vi "p2.vi"() -> ()   [LabVIEW 2023, in "d12.lvlib"]
uses:
  d12.lvlib
  AOC/AOC.lvlib
panel:
  out "Answer":u64=7670
  in  "Example":string="???.### 1,1,3\n.??..??...?##. 1,1,3\n?#?#?#?#?#?#?#? 1,3,1,6\n????.#...#... 4,1,1\n????.######..#####. 1,6,5\n?###???????? 3,2,1"
  in  "Example":bool
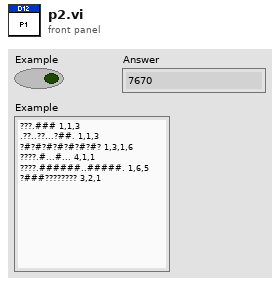
[diagram p1: front panel]
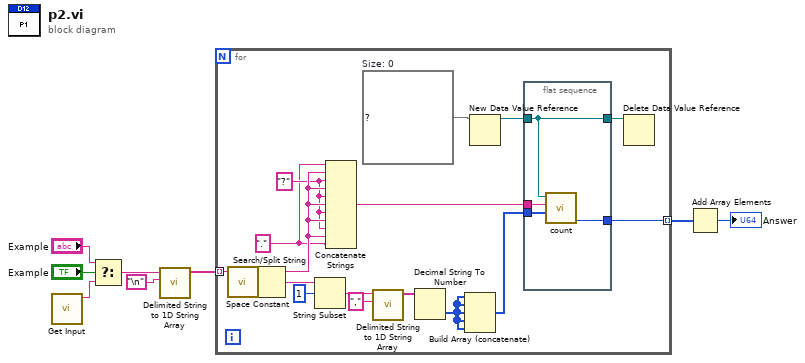
[diagram p0: block diagram]
diagram:
  n1 = call "Get Input.vi"() -> ("Input"=w8:string)  [unwired: 11 in]
  n2 = Select(t="Example", s="Example", f=w8) -> (s? t:f=w7:string)
  n3 = call <vilib>:"Delimited String to 1D String Array.vi"("delimiter"="\n", "delimited string"=w7) -> ("string array"=w3:string[])  [unwired: 9 in]
  n4 = for {
    tunnel: w3 -> [w25] mode=indexing
    tunnel: [w11] -> w1 mode=indexing
    w14 = map{cluster{string, "nums":i32[]}, u64} {}  # Size: 0
    w17 = "." ("string")
    w18 = "?" ("string")
    n5 = call <vilib>:"Space Constant.vi"() -> ("String"=w24:string)
    n6 = Search/Split String(string=w25, search string/char (-)=w24) -> (substring before match=w19:string, match + rest of string=w23:string)  [unwired: 1 in, 1 out]
    n7 = String Subset(string=w23, offset (0)=1) -> (substring=w21:string)  [unwired: 1 in]
    n8 = Concatenate Strings(w17, w19, w18, w19, w18, w19, w18, w19, w18, w19, w17) -> (w13:string)
    n9 = call <vilib>:"Delimited String to 1D String Array.vi"("delimiter"=",", "delimited string"=w21) -> ("string array"=w16:string[])  [unwired: 9 in]
    n10 = Decimal String To Number(string=w16) -> (number=w15:i32[])  [unwired: 2 in, 1 out]
    n11 = Build Array (concatenate)(w15, w15, w15, w15, w15) -> (w12:i32[])
    n12 = New Data Value Reference(data value=w14) -> (data value reference=w10:refnum<data-value>)  [unwired: 1 in, 1 out]
    n13 = flat-sequence {
      tunnel: w13 -> [w29]
      tunnel: w12 -> [w28]
      tunnel: [w27] -> w11
      tunnel: w10 -> [w26]
      tunnel: [w26] -> w9
      frame #0 {
        n14 = call "count.vi"("nums"=w28, "cfg"=w29, "cache"=w26) -> ("count"=w27:u64)  [unwired: 8 in]
      }
    }
    n15 = Delete Data Value Reference(data value reference=w9) -> ()  [unwired: 1 in, 2 out]
  }
  n16 = Add Array Elements(numeric array=w1) -> (sum=→"Answer":u64)
